vi "AnalogTrigger.vi"(1 "EdgeType":i32, 2 "TriggerLevel":sgl, 3 "AnalogChannel":refnum<k24>, 4 "SmartScope in":refnum<k24>) -> (0 "SmartScope out":refnum<k24>)   [LabVIEW 2013]
uses:
  C:/Program Files (x86)/LabNation/SmartScope/DeviceInterface.dll
  Program Files (x86)/LabNation/SmartScope/DeviceInterface.dll
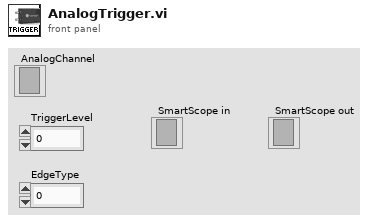
[diagram p1: front panel]
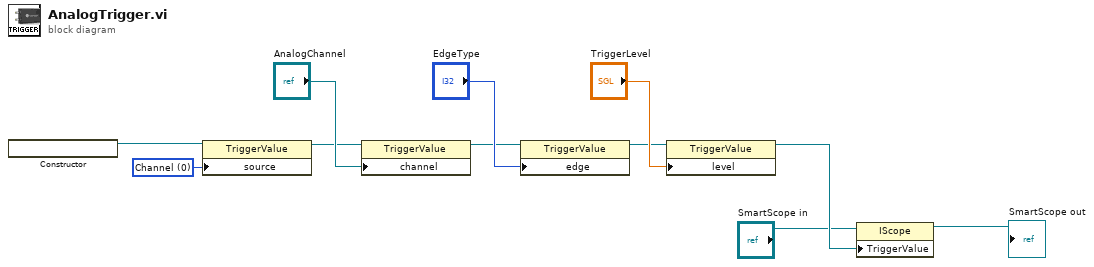
[diagram p0: block diagram]
diagram:
  w5 = 0 items=["Channel", "External"] ("source")
  n1 = constructor class="TriggerValue"() -> (reference out=w4:refnum<k24>)  [unwired: 3 in, 2 out]
  n2 = property class="TriggerValue"(reference=w4, "source"=w5) -> (reference out=w6:refnum<k24>)  [unwired: 1 in, 1 out]
  n3 = property class="TriggerValue"(reference=w6, "channel"="AnalogChannel") -> (reference out=w8:refnum<k24>)  [unwired: 1 in, 1 out]
  n4 = property class="TriggerValue"(reference=w8, "edge"="EdgeType") -> (reference out=w10:refnum<k24>)  [unwired: 1 in, 1 out]
  n5 = property class="TriggerValue"(reference=w10, "level"="TriggerLevel") -> (reference out=w3:refnum<k24>)  [unwired: 1 in, 1 out]
  n6 = property class="IScope"(reference="SmartScope in", "TriggerValue"=w3) -> (reference out=→"SmartScope out":refnum<k24>)  [unwired: 1 in, 1 out]
